vi "dynanometer.vi"() -> ()   [LabVIEW 2013]
uses:
  <vilib>/Instr/_visa.llb/VISA Configure Serial Port (Instr).vi
panel:
  out "CVT Ratio":dbl(knob) scale=0.0..3600.0
  out "CVT Ratio":dbl
  out "Engine Power (kW)":dbl(knob) scale=0.0..3600.0
  out "Engine Power (kW)":dbl
  in  "Tare":bool
  in  "Set CVT Position":bool
  out "Output to TSC":string
  in  "Target CVT  Position":dbl(knob) scale=0.0..255.0
  out "Engine Torque (Nm)":dbl
  out "Engine Torque (Nm)":dbl(knob) scale=0.0..10.0
  in  "Load Cell Port":refnum<visa-resource-name>
  out "CVT Target":dbl(slide) scale=0.0..255.0
  out "CVT Position":dbl(slide) scale=0.0..255.0
  out "Wheel RPM":dbl(knob) scale=0.0..1000.0
  out "Engine (Primary) RPM":dbl(knob) scale=0.0..3600.0
  out "Driveshaft (Secondary) RPM":dbl(knob) scale=0.0..10000.0
  out "Checksum OK":bool
  out "data":T1
  out "String":string
  out "Checksum":i32
  in  "stop":bool
  in  "Baud Rate (9600)":u32=9600
  in  "TSC Port":refnum<visa-resource-name>
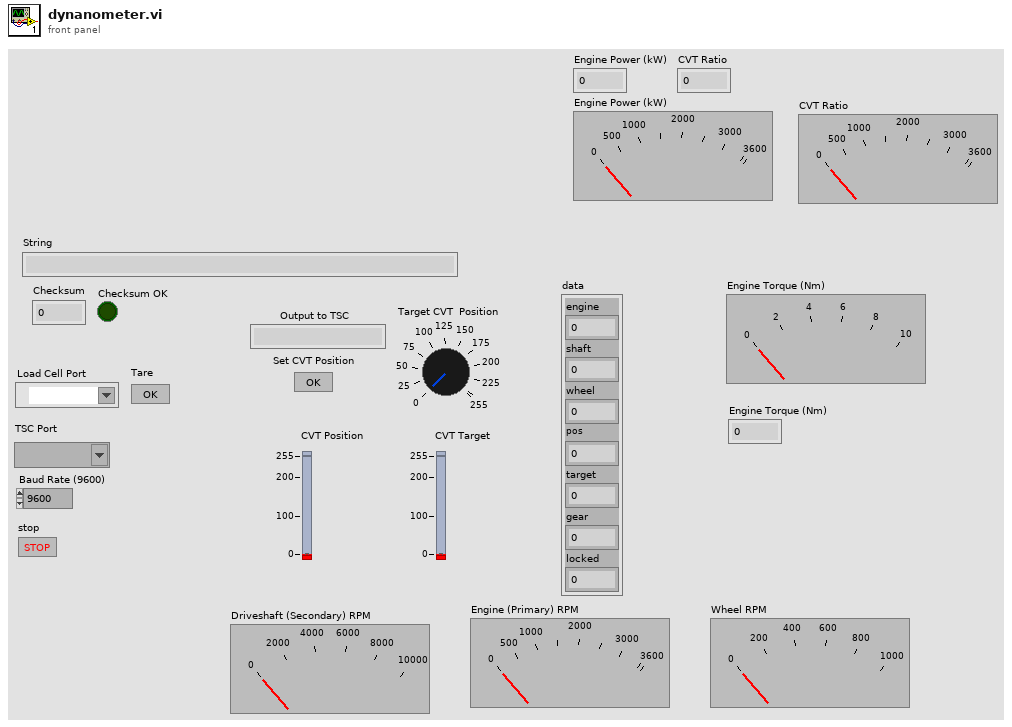
[diagram p1: front panel]
types:
  T1 = cluster{"engine":i32, "shaft":i32, "wheel":i32, "pos":i32, "target":i32, "gear":i32, "locked":i32}
  T2 = enum16{"open", "replace", "create", "open or create", "replace or create", "replace or create with confirmation"}
  T3 = cluster{"data":cluster{"engine":i32, "shaft":i32, "wheel":i32, "pos":i32, "target":i32, "gear":i32, "locked":i32}, "chksum":i32}
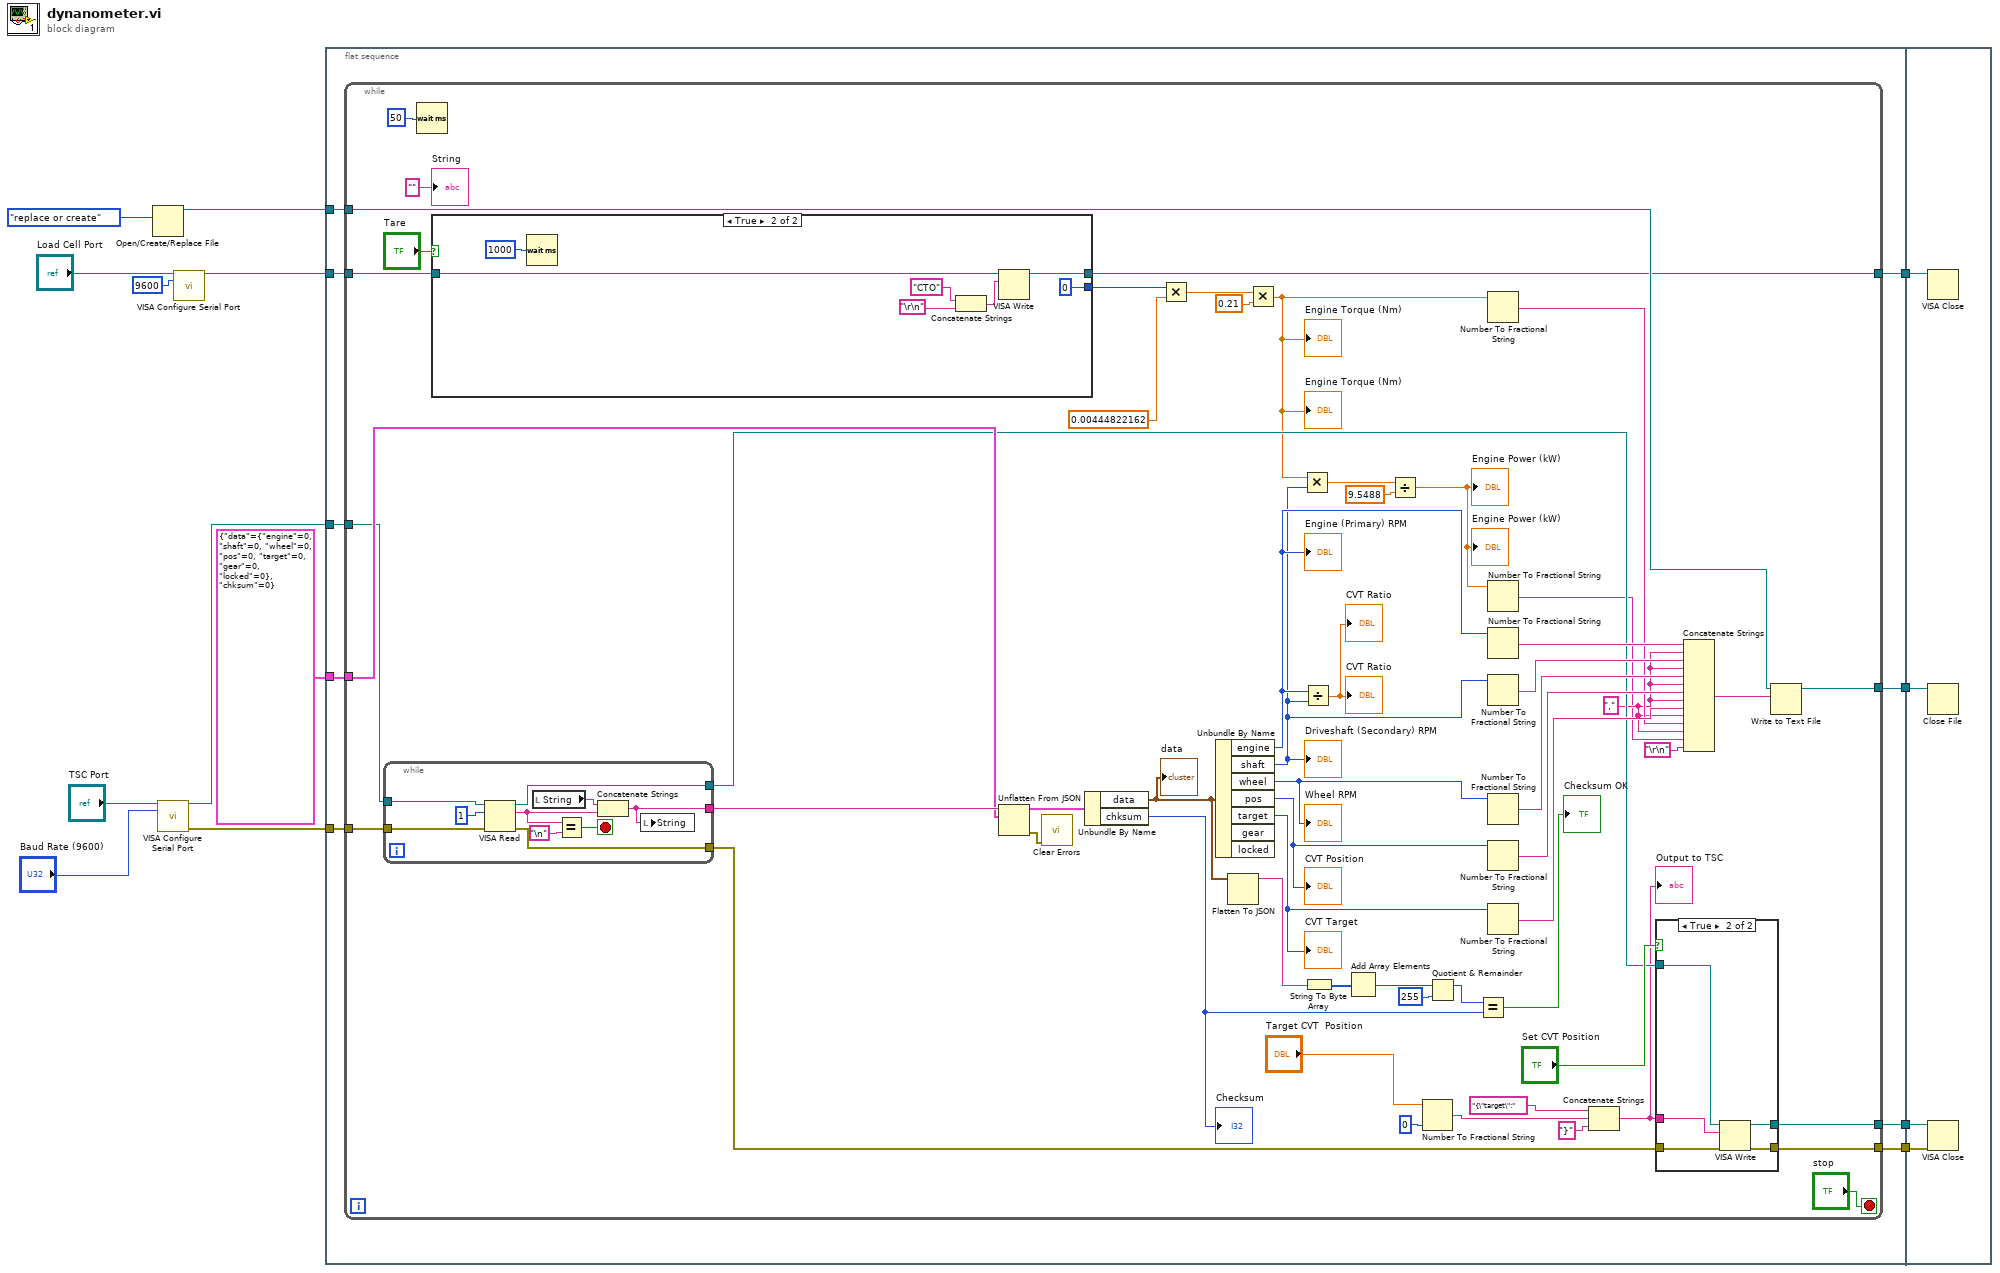
[diagram p0: block diagram]
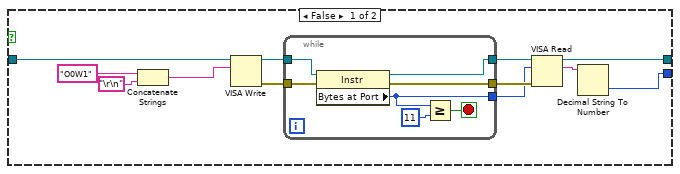
[diagram p2: hidden frame]
diagram:
  n1 = Open/Create/Replace File(operation (0:open)=T2."replace or create") -> (refnum out=w9:refnum<file>)  [unwired: 5 in, 2 out]
  n2 = call-poly "VISA Configure Serial Port"("VISA resource name"="TSC Port", "baud rate (9600)"="Baud Rate (9600)") -> ("VISA resource name out"=w13:refnum<visa-resource-name>, "error out"=w2:errorcluster)  [unwired: 12 in]
  n3 = call-poly "VISA Configure Serial Port"("VISA resource name"="Load Cell Port", "baud rate (9600)"=u32 9600) -> ("VISA resource name out"=w3:refnum<visa-resource-name>)  [unwired: 12 in, 1 out]
  n4 = flat-sequence {
    tunnel: w13 -> [w23]
    tunnel: T3 {"data"={"engine"=0, "shaft"=0, "wheel"=0, "pos"=0, "target"=0, "gear"=0, "locked"=0}, "chksum"=0} ("type and defaults") -> [w22]
    tunnel: [w21] -> w10
    tunnel: w9 -> [w20]
    tunnel: [w19] -> w8
    tunnel: [w18] -> w5
    tunnel: w3 -> [w17]
    tunnel: w2 -> [w16]
    tunnel: [w15] -> w1
    tunnel: w10 -> [w127]
    tunnel: w8 -> [w126]
    tunnel: w5 -> [w125]
    tunnel: w1 -> [w124]
    frame #0 {
      n5 = while {
        tunnel: w23 -> [w69]
        tunnel: w22 -> [w76]
        tunnel: [w37] -> w21
        tunnel: w20 -> [w65]
        tunnel: [w64] -> w19
        tunnel: [w50] -> w18
        tunnel: w17 -> [w49]
        tunnel: w16 -> [w42]
        tunnel: [w38] -> w15
        stop <- "stop" stop-if-true
        w28 = ","
        n6 = while {
          tunnel: w69 -> [w123]
          tunnel: [w122] -> w40
          tunnel: [w116] -> w79
          tunnel: w42 -> [w115]
          tunnel: [w114] -> w39
          stop <- w119 stop-if-true
          n7 = VISA Read(VISA resource name=w123, byte count=u32 1, error in (no error)=w115) -> (VISA resource name out=w122:refnum<visa-resource-name>, read buffer=w121:string, error out=w114:errorcluster)  [unwired: 1 out]
          n8 = local read "String"() -> (w117:string)
          n9 = Equal?(x=w121, y="\n") -> (x = y?=w119:bool)
          n10 = Concatenate Strings(w117, w121) -> (w116:string)
          n11 = local write "String"(w116) -> ()
        }
        n12 = Wait (ms)(milliseconds to wait=u32 50) -> ()  [unwired: 1 out]
        n13 = case shown="True" "Tare" {
          tunnel: [w90 w102] -> w50
          tunnel: w49 -> [w86 w103]
          tunnel: [w81 0] -> w34
          frame False {
            n14 = Concatenate Strings("O0W1" ("write buffer"), "\r\n") -> (w83:string)
            n15 = VISA Write(VISA resource name=w86, write buffer=w83) -> (VISA resource name out=w85:refnum<visa-resource-name>, error out=w84:errorcluster)  [unwired: 1 in, 1 out]
            n16 = while {
              tunnel: [w99] -> w92
              tunnel: [w97] -> w91
              tunnel: [w95] -> w89
              tunnel: w85 -> [w94]
              tunnel: w84 -> [w93]
              stop <- w98 stop-if-true
              n17 = property class="Instr"(reference=w94, error in=w93) -> (reference out=w99:refnum<visa-resource-name>, error out=w97:errorcluster, "Bytes at Port"=w95:u32)
              n18 = Greater Or Equal?(x=w95, y=u32 11) -> (x >= y?=w98:bool)
            }
            n19 = VISA Read(VISA resource name=w92, byte count=w89, error in (no error)=w91) -> (VISA resource name out=w90:refnum<visa-resource-name>, read buffer=w82:string)  [unwired: 2 out]
            n20 = Decimal String To Number(string=w82) -> (number=w81:i32)  [unwired: 2 in, 1 out]
          }
          frame True {
            n21 = Wait (ms)(milliseconds to wait=u32 1000) -> ()  [unwired: 1 out]
            n22 = Concatenate Strings("CTO" ("write buffer"), "\r\n") -> (w104:string)
            n23 = VISA Write(VISA resource name=w103, write buffer=w104) -> (VISA resource name out=w102:refnum<visa-resource-name>)  [unwired: 1 in, 2 out]
          }
        }
        n24 = Unflatten From JSON(JSON string=w79, type and defaults=w76) -> (value=w68:T3, error out=w78:errorcluster)  [unwired: 5 in]
        n25 = call <vilib>:"Clear Errors.vi"("error in (no error)"=w78) -> ()  [unwired: 6 in, 1 out]
        n26 = Unbundle By Name(w68) -> ("data"=w67:T1, "chksum"=w66:i32)
        "Checksum" <- w66
        "data" <- w67
        n27 = Multiply(x=w34, y=0.00444822162) -> (x*y=w53:dbl)
        n28 = Unbundle By Name(w67) -> ("engine"=w26:i32, "shaft"=w25:i32, "wheel"=w61:i32, "pos"=w59:i32, "target"=w58:i32)  [unwired: 2 out]
        "Driveshaft (Secondary) RPM" <- w25
        "Engine (Primary) RPM" <- w26
        "Wheel RPM" <- w61
        "CVT Target" <- w58
        "CVT Position" <- w59
        n29 = Flatten To JSON(anything=w67) -> (JSON string=w75:string)  [unwired: 2 in, 1 out]
        n30 = Multiply(x=w53, y=0.21) -> (x*y=w32:dbl)
        "Engine Torque (Nm)" <- w32
        "Engine Torque (Nm)" <- w32
        n31 = Multiply(x=w32, y=w25) -> (x*y=w31:dbl)
        n32 = Divide(x=w26, y=w25) -> (x/y=→"CVT Ratio" →"CVT Ratio":dbl)
        n33 = String To Byte Array(string=w75) -> (unsigned byte array=w74:u8[])
        n34 = Add Array Elements(numeric array=w74) -> (sum=w73:u8)
        n35 = Divide(x=w31, y=9.5488) -> (x/y=w29:dbl)
        "Engine Power (kW)" <- w29
        "Engine Power (kW)" <- w29
        n36 = Number To Fractional String(number="Target CVT  Position", precision (6)=i16 0) -> (F-format string=w43:string)  [unwired: 2 in]
        n37 = Quotient & Remainder(x=w73, y=u8 255) -> (x-y*floor(x/y)=w71:u8)  [unwired: 1 out]
        n38 = Equal?(x=w71, y=w66) -> (x = y?=→"Checksum OK":bool)
        n39 = Number To Fractional String(number=w32) -> (F-format string=w51:string)  [unwired: 3 in]
        n40 = Number To Fractional String(number=w29) -> (F-format string=w27:string)  [unwired: 3 in]
        n41 = Number To Fractional String(number=w26) -> (F-format string=w63:string)  [unwired: 3 in]
        n42 = Number To Fractional String(number=w25) -> (F-format string=w62:string)  [unwired: 3 in]
        n43 = Number To Fractional String(number=w61) -> (F-format string=w60:string)  [unwired: 3 in]
        n44 = Number To Fractional String(number=w59) -> (F-format string=w57:string)  [unwired: 3 in]
        n45 = Number To Fractional String(number=w58) -> (F-format string=w56:string)  [unwired: 3 in]
        n46 = Concatenate Strings("{\"target\":", w43, "}") -> (w36:string)
        "Output to TSC" <- w36
        n47 = case shown="True" "Set CVT Position" {
          tunnel: w40 -> [w108 w113]
          tunnel: w39 -> [w107 w112]
          tunnel: [w107 w111] -> w38
          tunnel: [w108 w110] -> w37
          tunnel: w36 -> [_ w109]
          frame False {
          }
          frame True {
            n48 = VISA Write(VISA resource name=w113, write buffer=w109, error in (no error)=w112) -> (VISA resource name out=w110:refnum<visa-resource-name>, error out=w111:errorcluster)  [unwired: 1 out]
          }
        }
        n49 = Concatenate Strings(w63, w28, w62, w28, w60, w28, w57, w28, w56, w28, w51, w28, w27, "\r\n") -> (w55:string)
        n50 = Write to Text File(file (use dialog)=w65, text=w55) -> (refnum out=w64:refnum<file>)  [unwired: 2 in, 2 out]
        "String" <- ""
      }
    }
    frame #1 {
      n51 = VISA Close(VISA resource name=w125) -> ()  [unwired: 1 in, 1 out]
      n52 = Close File(refnum=w126) -> ()  [unwired: 1 in, 2 out]
      n53 = VISA Close(VISA resource name=w127, error in (no error)=w124) -> ()  [unwired: 1 out]
    }
  }
